vi "Add FIU Card From Table.vi"(8 "error in (no error)":errorcluster, 10 "Card Position":T1={"Rack #"=0, "Slot #"=1} {"Slot #" max=15}, 11 "Node Ptr":u64 format="%.0x") -> (0 "error out":errorcluster)   [LabVIEW 2014, in "SLSC configuration System Explorer.lvlib"]
uses:
  SLSC configuration System Explorer.lvlib
  Type Defs/Card Position.ctl
  Example/SPI Utility/Slot #.ctl
  <vilib>/NI Veristand/Custom Device API/Custom Device Channel.ctl
  <vilib>/NI Veristand/Custom Device API/Custom Device Channel Type.ctl
  Shared/Constants.vi
  <vilib>/NI Veristand/Custom Device API/Set Item Property (U16).vi
  Shared/SLSC configuration Shared.lvlib
  <vilib>/NI Veristand/Custom Device API/Custom Device API.lvlib
  <vilib>/NI Veristand/Custom Device Tools/Custom Device Utility Library/Custom Device Utility Library.lvlib
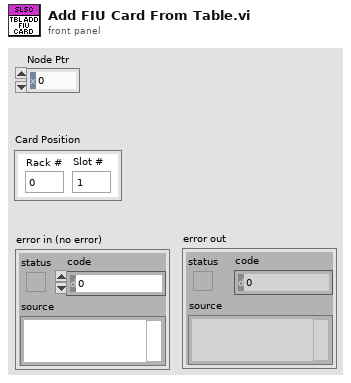
[diagram p1: front panel]
types:
  T1 = typedef "SLSC configuration Shared.lvlib/Card Position.ctl" = cluster{"Rack #":u8, "Slot #":T2}
  T2 = typedef "SLSC configuration Shared.lvlib/Slot #.ctl" = u8
  T3 = typedef "Custom Device API.lvlib/Custom Device Channel Type.ctl" = enum16{"Input", "Output"}
  T4 = typedef "Custom Device API.lvlib/Custom Device Channel.ctl" = cluster{"Type":T3, "Units":string, "Default Value":dbl, "Faultable":bool, "Scalable":bool}
  T5 = typedef "Custom Device API.lvlib/Custom Device Item Ref.ctl" = u64
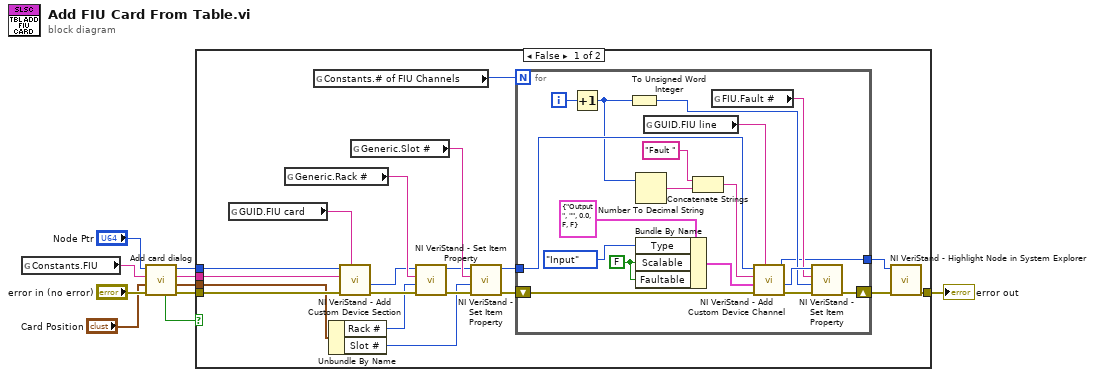
[diagram p0: block diagram]
diagram:
  n1 = global read "Constants.vi" "Constants.FIU"() -> (w4:string)
  n2 = call "Add card dialog.vi"("error in (no error)"="error in (no error)", "Card Position"="Card Position", "Card Type in"=w4, "Node Ptr"="Node Ptr") -> ("error out"=w8:errorcluster, "Card Position out"=w5:cluster{"Rack #":u8, "Slot #":T2}, "Name out"=w9:string, "Node Ptr out"=w10:u64, "Cancelled?"=w1:bool)  [unwired: 3 in]
  n3 = case shown="False" w1 {
    tunnel: w10 -> [w29 _]
    tunnel: w9 -> [w28 _]
    tunnel: w8 -> [w27 w48]
    tunnel: w5 -> [w19 _]
    tunnel: [w12 w48] -> w3
    frame False {
      n4 = global read "Constants.vi" "GUID.FIU card"() -> (w26:string)
      n5 = global read "Constants.vi" "Generic.Rack #"() -> (w25:string)
      n6 = global read "Constants.vi" "Constants.# of FIU Channels"() -> (w11:u8)
      n7 = Unbundle By Name(w19) -> ("Rack #"=w15:u8, "Slot #"=w21:T2)
      n8 = call <vilib>:"NI VeriStand - Add Custom Device Section.vi"("GUID (Default Section)"=w26, "error in (no error)"=w27, "Section Name"=w28, "Parent Ref in"=w29) -> ("error out"=w20:errorcluster, "Section Ptr"=w16:T5)  [unwired: 4 in, 2 out]
      n9 = global read "Constants.vi" "Generic.Slot #"() -> (w23:string)
      n10 = call-poly <vilib>:"NI VeriStand - Set Item Property.vi"("error in (no error)"=w20, "Value"=w15, "Property Name"=w25, "Item Ref in"=w16) -> ("error out"=w24:errorcluster, "Item Ref out"=w22:T5)  [unwired: 5 in, 1 out]
      n11 = call-poly <vilib>:"NI VeriStand - Set Item Property.vi"("error in (no error)"=w24, "Value"=w21, "Property Name"=w23, "Item Ref in"=w22) -> ("error out"=w18:errorcluster, "Item Ref out"=w17:T5)  [unwired: 5 in, 1 out]
      n12 = for {
        N: w11 -> [_]
        shift-right: [w39] -> w14
        shift-left: w18 -> [w45]
        tunnel: w17 -> [w46]
        tunnel: [w30] -> w13
        i -> [w47]
        w31 = FALSE ("Scalable")
        n13 = Increment(x=w47) -> (x+1=w36:i32)
        n14 = To Unsigned Word Integer(number=w36) -> (unsigned 16bit integer=w35:u16)
        n15 = Number To Decimal String(number=w36) -> (decimal integer string=w43:string)  [unwired: 1 in]
        n16 = Bundle By Name(cluster=T4 {"Type"=enum."Output", "Units"="", "Default Value"=0.0, "Faultable"=FALSE, "Scalable"=FALSE} ("Channel"), "Type"=Custom_Device_Channel_Type."Input", "Scalable"=w31, "Faultable"=w31) -> (w33:T4)
        n17 = global read "Constants.vi" "GUID.FIU line"() -> (w44:string)
        n18 = Concatenate Strings("Fault " ("Channel Name"), w43) -> (w41:string)
        n19 = global read "Constants.vi" "FIU.Fault #"() -> (w37:string)
        n20 = call <vilib>:"NI VeriStand - Add Custom Device Channel.vi"("GUID (Default Channel)"=w44, "error in (no error)"=w45, "Channel"=w33, "Channel Name"=w41, "Parent Ref in"=w46) -> ("error out"=w40:errorcluster, "Channel Ref"=w38:T5, "Parent Ref out"=w30:T5)  [unwired: 3 in, 1 out]
        n21 = call-poly <vilib>:"NI VeriStand - Set Item Property.vi"("error in (no error)"=w40, "Value"=w35, "Property Name"=w37, "Item Ref in"=w38) -> ("error out"=w39:errorcluster)  [unwired: 5 in, 2 out]
      }
      n22 = call <vilib>:"NI VeriStand - Highlight Node in System Explorer.vi"("error in (no error)"=w14, "Item Ref in"=w13) -> ("error out"=w12:errorcluster)  [unwired: 8 in, 1 out]
    }
    frame True {
    }
  }
  "error out" <- w3
